vi "Remote.TCP-IP Listener.vi"(8 "StatusCtrlRef":refnum<vi>, 9 "Main Q In":refnum<queue>, 10 "Config Folder":path, 11 "Q Name":string="Remote") -> ()   [LabVIEW 2018]
uses:
  <vilib>/KATE/Queues/Queue Utils.lvlib
  <vilib>/KATE/TCP-IP/TCP-IP.lvlib
  <vilib>/KATE/TCP-IP/Link/Controls/TCP-IP Link.Config.ctl
  <vilib>/KATE/TCP-IP/Link/Controls/TCP-IP Link.Packet Format.ctl
  <vilib>/KATE/TCP-IP/Link/Controls/TCP-IP Link.Options.ctl
  <vilib>/KATE/Queues/Q.Element.ctl
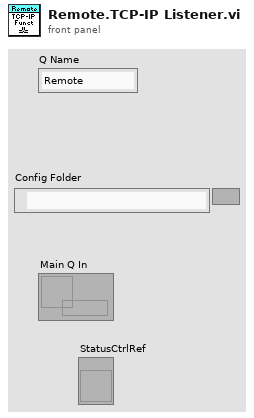
[diagram p1: front panel]
types:
  T1 = typedef "TCP-IP.lvlib/TCP-IP Link.Packet Format.ctl" = enum16{"First 2 Bytes is Length (U16)", "First 3 Chars is Length"}
  T2 = typedef "KATE_Lib.lvlib/Queue Utils.lvlib/Q.Element.ctl" = cluster{"Cmd":string, "Sub":string, "Data1":variant, "Data2":variant}
  T3 = typedef "KATE_Lib.lvlib/TCP-IP.lvlib/TCP-IP Link.Options.ctl" = cluster{"Status Notify En":bool, "Auto Connect":bool, "Packet Format":T4}
  T4 = typedef "KATE_Lib.lvlib/TCP-IP.lvlib/TCP-IP Link.Packet Format.ctl" = enum16{"First 2 Bytes is Length (U16)", "First 3 Chars is Length"}
  T5 = typedef "KATE_Lib.lvlib/TCP-IP.lvlib/TCP-IP Link.Config.ctl" = cluster{"IP":string, "Port":u16, "Listener":bool}
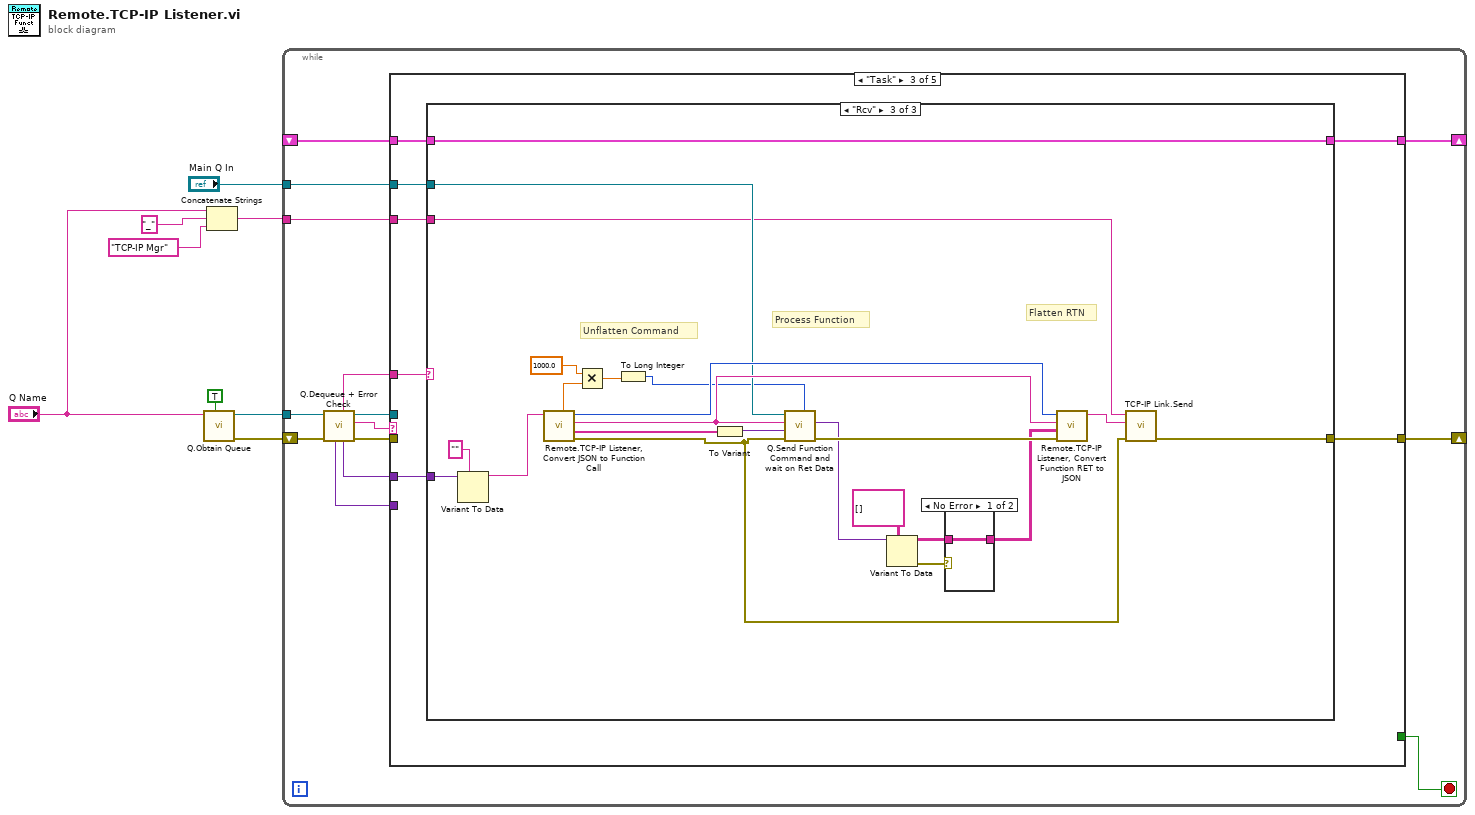
[diagram p0: block diagram]
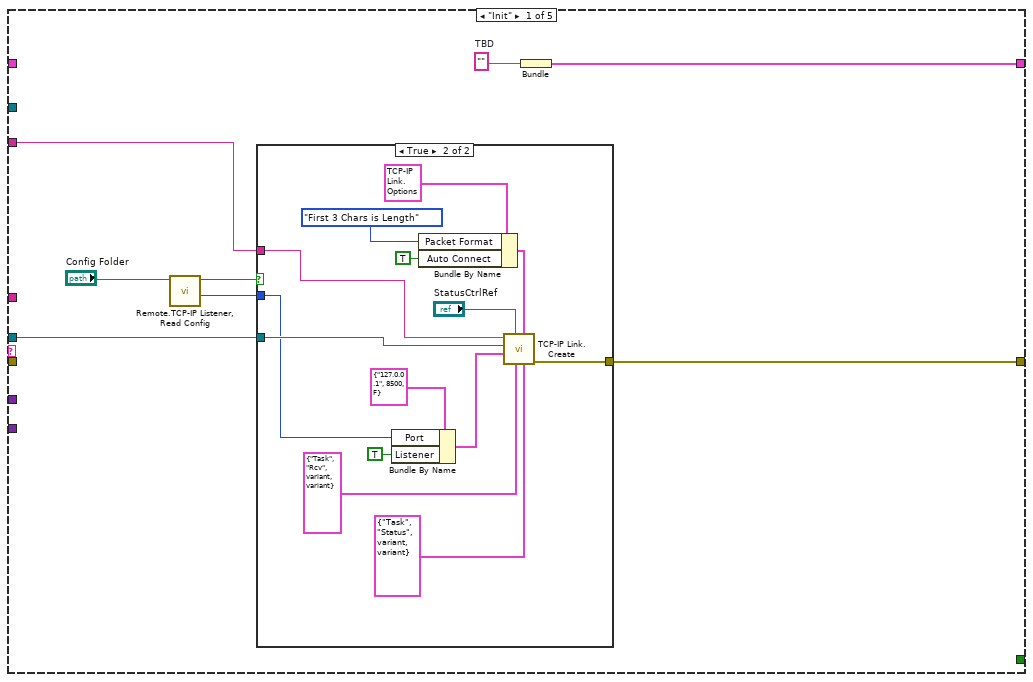
[diagram p2: hidden frame]
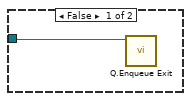
[diagram p3: hidden frame]
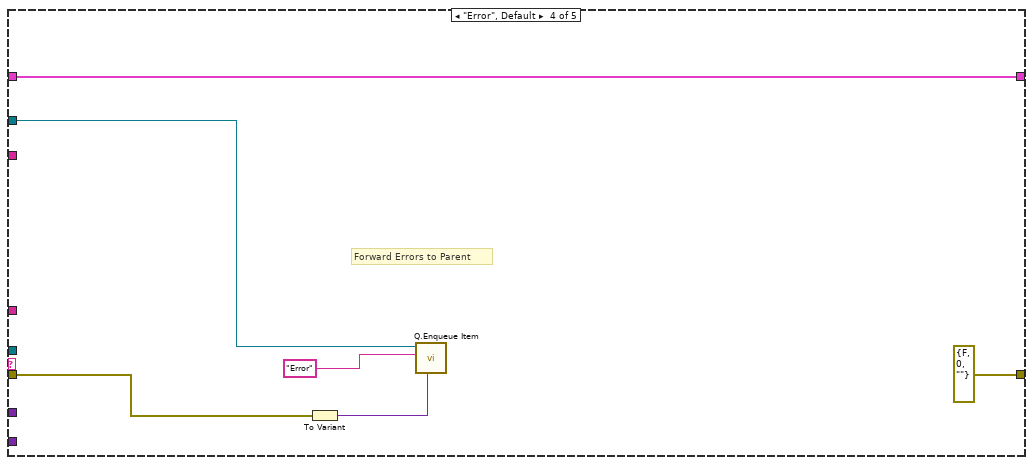
[diagram p8: hidden frame]
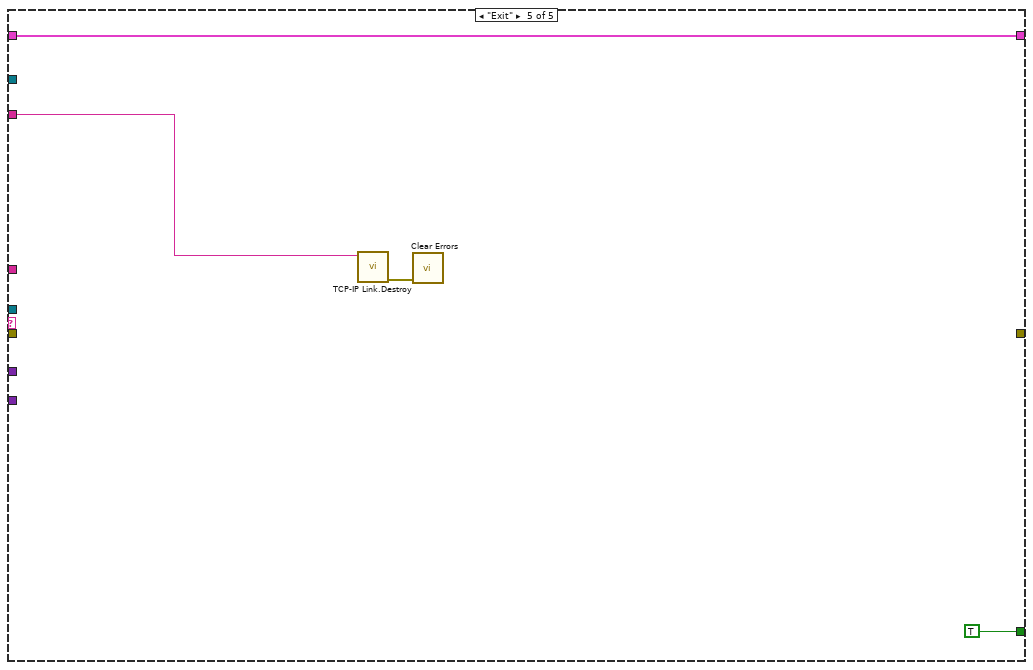
[diagram p9: hidden frame]
diagram:
  n1 = call <vilib>:"Q.Obtain Queue.vi"("Enqueue Init"=TRUE, "Q Name"="Q Name") -> ("error out"=w6:errorcluster, "Q Out"=w8:refnum<queue>)  [unwired: 7 in, 1 out]
  n2 = Concatenate Strings("Q Name", "_" ("string"), "TCP-IP Mgr" ("Q Name")) -> (w1:string)
  n3 = while {
    tunnel: w8 -> [w22]
    shift-right: [w13] -> _
    shift-left: w6 -> [w18]
    tunnel: "Main Q In" -> [w14]
    shift-right: [w10] -> _
    shift-left: _ -> [w11]
    tunnel: w1 -> [w9]
    stop <- w12 stop-if-true
    n4 = call <vilib>:"Q.Dequeue + Error Check.vi"("Error In"=w18, "Q In"=w22) -> ("error out"=w19:errorcluster, "Cmd"=w20:string, "Q Out"=w21:refnum<queue>, "Data1"=w17:variant, "Sub"=w15:string, "Data2"=w16:variant)  [unwired: 4 in]
    n5 = case shown="\"Task\"" w20 {
      tunnel: w21 -> [w30 _ _ _ _]
      tunnel: w19 -> [_ _ _ w83 _]
      tunnel: w17 -> [_ _ w49 _ _]
      tunnel: w16 -> [_ _ _ _ _]
      tunnel: w15 -> [_ _ w51 _ _]
      tunnel: w14 -> [_ _ w50 w85 _]
      tunnel: [w27 _ w47 errorcluster {"status"=FALSE, "code"=0, "source"=""} ("error constant") _] -> w13
      tunnel: [_ _ _ _ TRUE] -> w12
      tunnel: w11 -> [_ w46 w52 w80 w87]
      tunnel: [w23 w46 w53 w80 w87] -> w10
      tunnel: w9 -> [w29 _ w48 _ w86]
      frame "Init" {
        w24 = ""  # TBD
        n6 = call "Remote.TCP-IP Listener, Read Config.vi"("Config Folder"="Config Folder") -> ("Port"=w25:i32, "Enabled"=w26:bool)  [unwired: 9 in]
        n7 = case shown="True" w26 {
          tunnel: w30 -> [w31 w45]
          tunnel: w29 -> [_ w44]
          tunnel: [_ w38] -> w27
          tunnel: w25 -> [_ w42]
          frame False {
            n8 = call <vilib>:"Q.Enqueue Exit.vi"("Q In"=w31) -> ()  [unwired: 9 in, 2 out]
          }
          frame True {
            n9 = Bundle By Name(cluster=T5 {"IP"="127.0.0.1", "Port"=8500, "Listener"=FALSE} ("Config"), "Port"=w42, "Listener"=TRUE) -> (w32:T5)
            n10 = Bundle By Name(cluster=T3 {"Status Notify En"=TRUE, "Auto Connect"=TRUE, "Packet Format"=enum."First 2 Bytes is Length (U16)"} ("Options"), "Packet Format"=TCP-IP_Link.Packet_Format."First 3 Chars is Length", "Auto Connect"=TRUE) -> (w34:T3)
            n11 = call <vilib>:"TCP-IP Link.Create.vi"("Status Element"=T2 {"Cmd"="Task", "Sub"="Status", "Data1"=variant, "Data2"=variant}, "Options"=w34, "Rcv Data Element"=T2 {"Cmd"="Task", "Sub"="Rcv", "Data1"=variant, "Data2"=variant}, "StatusCtrlRef"="StatusCtrlRef", "Config"=w32, "Q_RcvData"=w45, "Control Q Name"=w44) -> ("Error Out"=w38:errorcluster)  [unwired: 3 in, 1 out]
          }
        }
        n12 = Bundle("TBD"=w24) -> (w23:cluster{"TBD":string})  [unwired: 1 in]
      }
      frame "Reset" {
      }
      frame "Task" {
        n13 = case shown="\"Rcv\"" w51 {
          tunnel: [w54 w55 w78] -> w53
          tunnel: w52 -> [w54 w55 w78]
          tunnel: w50 -> [_ _ w73]
          tunnel: w49 -> [_ _ w66]
          tunnel: w48 -> [_ _ w63]
          tunnel: [_ _ w60] -> w47
          frame Default {
          }
          frame "Status" {
          }
          frame "Rcv" {
            # "Process Function"
            # "Flatten RTN"
            # "Unflatten Command"
            n14 = Variant To Data(type="", Variant=w66) -> (data=w64:string)  [unwired: 1 in, 1 out]
            n15 = call "Remote.TCP-IP Listener, Convert JSON to Function Call.vi"("JSON"=w64) -> ("error out"=w61:errorcluster, "Args"=w76:string[], "Function"=w74:string, "Seq"=w77:i32, "Timeout"=w59:dbl)  [unwired: 6 in]
            n16 = Multiply(x=1000.0, y=w59) -> (x*y=w57:dbl)
            n17 = To Long Integer(number=w57) -> (32bit integer=w56:i32)
            n18 = To Variant(anything=w76) -> (Variant=w75:variant)
            n19 = call <vilib>:"Q.Send Function Command and wait on Ret Data.vi"("Timeout(ms)"=w56, "error in"=w61, "Data1"=w75, "Cmd"=w74, "Q In"=w73) -> ("error out"=w72:errorcluster, "Ret"=w70:variant)  [unwired: 5 in]
            n20 = Variant To Data(type=string[][] [], Variant=w70) -> (data=w68:string[][], error out=w69:errorcluster)  [unwired: 1 in]
            n21 = case shown="No Error" w69 {
              tunnel: w68 -> [w79 _]
              tunnel: [w79 _] -> w67
              frame No Error {
              }
              frame Error {
              }
            }
            n22 = call "Remote.TCP-IP Listener, Convert Function RET to JSON.vi"("Rtn Error"=w72, "Data"=w67, "Funct"=w74, "Seq"=w77) -> ("JSON"=w62:string)  [unwired: 7 in]
            n23 = call <vilib>:"TCP-IP Link.Send.vi"("error in"=w61, "Data"=w62, "Link Q Name"=w63) -> ("error out"=w60:errorcluster)  [unwired: 8 in]
          }
        }
      }
      frame "Error", Default {
        # "Forward Errors to Parent"
        n24 = To Variant(anything=w83) -> (Variant=w82:variant)
        n25 = call <vilib>:"Q.Enqueue Item.vi"("Data1"=w82, "Cmd"="Error", "Q In"=w85) -> ()  [unwired: 7 in, 2 out]
      }
      frame "Exit" {
        n26 = call <vilib>:"TCP-IP Link.Destroy.vi"("Q Name"=w86) -> ("error out"=w88:errorcluster)  [unwired: 10 in]
        n27 = call <vilib>:"Clear Errors.vi"("error in (no error)"=w88) -> ()  [unwired: 5 in, 2 out]
      }
    }
  }
